vi "ConfigInstr.vi"(6 "InstrumentName":string, 7 "VisaRessIn":refnum<visa-resource-name>, 8 "error in (no error)":errorcluster caption="entrée d'erreur (pas d'erreur)", 9 "FirstClassInst":bool, 10 "Function":string, 11 "GenData In":refnum<class "Monospec50.lvclass"> caption="DNL_LabVIEW Object in") -> (0 "error out":errorcluster caption="sortie d'erreur", 3 "GenData Out":refnum<class "Monospec50.lvclass"> caption="DNL_LabVIEW Object out")   [LabVIEW 2012, in "Monospec50.lvclass"]
uses:
  Monospec50.lvclass
  Monospec50_Func.ctl
  Monospec50.lvclass/Monospec50.ctl
  BaseDevice/BaseDevice.lvclass/BaseDevice.ctl
  BaseDevice/Accessor/SetShowInstrNm.vi
panel:
  in  "Class_Func":T1
  out "VisaRessOut":refnum<visa-resource-name>
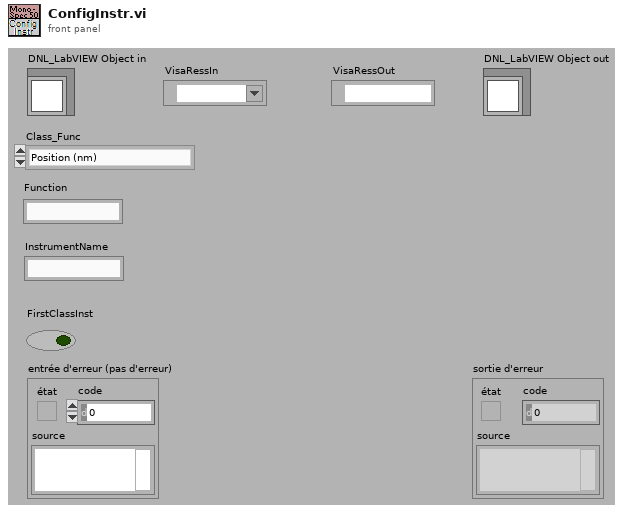
[diagram p1: front panel]
types:
  T1 = typedef "Monospec50.lvclass/Monospec50_Func.ctl" = enum16{"Position (nm)"}
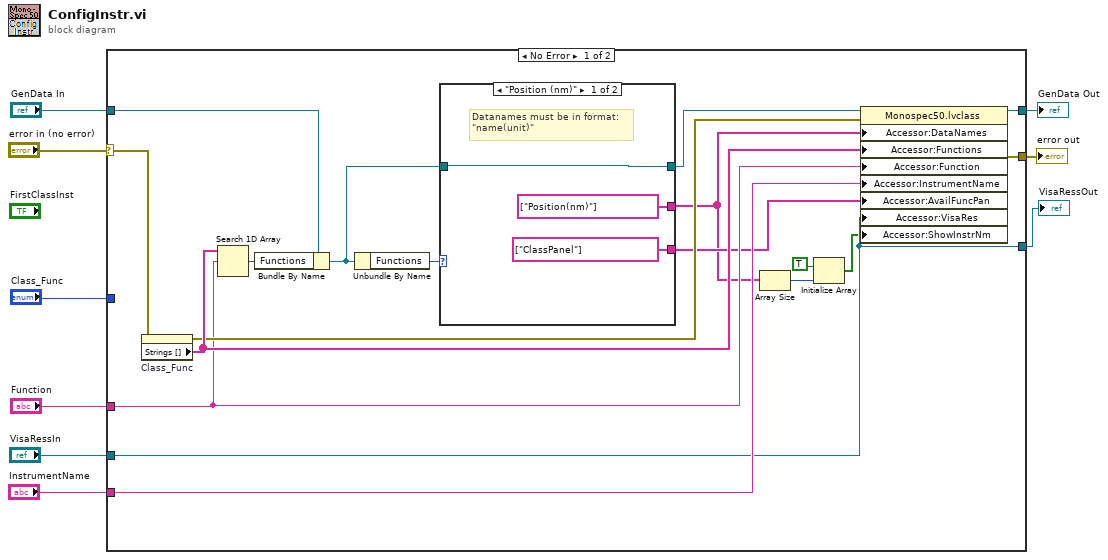
[diagram p0: block diagram]
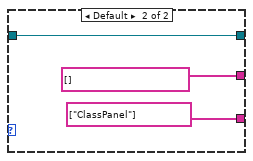
[diagram p2: hidden frame]
diagram:
  n1 = case shown="No Error" "error in (no error)" {
    selector: "error in (no error)" -> [w21 w35]
    tunnel: [w27 w35] -> w8
    tunnel: "GenData In" -> [w22 w34]
    tunnel: [w26 w34] -> w6
    tunnel: "Class_Func" -> [_ _]
    tunnel: "Function" -> [w17 _]
    tunnel: "InstrumentName" -> [w16 _]
    tunnel: "VisaRessIn" -> [w14 _]
    tunnel: [w14 _] -> w1
    frame No Error {
      n2 = property on="Class_Func" class="Enum (strict)"(error in=w21) -> (error out=w20:errorcluster, "Strings []"=w24:string[])  [unwired: 1 in, 1 out]
      n3 = Search 1D Array(1D array=w24, element=w17) -> (index of element=w23:i32)  [unwired: 1 in]
      n4 = Bundle By Name(cluster=w22, "Functions"=w23) -> (w19:refnum<class "Monospec50.lvclass">)
      n5 = Unbundle By Name(w19) -> ("Functions"=w25:T1)
      n6 = case shown="\"Position (nm)\"" w25 {
        tunnel: [string[] ["Position(nm)"] string[] []] -> w11
        tunnel: w19 -> [w30 w32]
        tunnel: [w30 w32] -> w18
        tunnel: [string[] ["ClassPanel"] string[] ["ClassPanel"]] -> w15
        frame "Position (nm)" {
          # "Datanames must be in format:\n\"name(unit)\""
        }
        frame Default {
        }
      }
      n7 = Array Size(array=w11) -> (size(s)=w13:i32)
      n8 = Initialize Array(TRUE, w13) -> (w10:bool[])
      n9 = property class="Monospec50.lvclass"(reference=w18, error in=w20, "Accessor:DataNames"=w11, "Accessor:Functions"=w24, "Accessor:Function"=w17, "Accessor:InstrumentName"=w16, "Accessor:AvailFuncPan"=w15, "Accessor:VisaRes"=w14, "Accessor:ShowInstrNm"=w10) -> (reference out=w26:refnum<class "Monospec50.lvclass">, error out=w27:errorcluster)
    }
    frame Error {
    }
  }
  "error out" <- w8
  "GenData Out" <- w6
  "VisaRessOut" <- w1
